vi "Number Generator.vi"() -> (3 "Random Number":i32)   [LabVIEW 2017]
doc: "Generates a valid number for the guessing game."
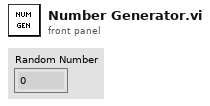
[diagram p1: front panel]
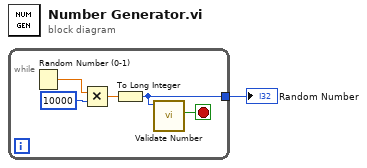
[diagram p0: block diagram]
diagram:
  n1 = while {
    tunnel: [w2] -> w1
    stop <- w6 stop-if-true
    n2 = Random Number (0-1)() -> (number: 0 to 1=w5:dbl)
    n3 = Multiply(x=w5, y=10000) -> (x*y=w3:dbl)
    n4 = To Long Integer(number=w3) -> (32bit integer=w2:i32)
    n5 = call "Validate Number.vi"("Number"=w2) -> ("Valid?"=w6:bool)  [unwired: 9 in, 1 out]
  }
  "Random Number" <- w1
